vi "TIO RPC Blocking.vi"(8 "error in (no error)":errorcluster, 9 "Payload":string, 10 "Named Method":string="mcu.desc", 11 "TS Connection":T1={"Type"=enum."TCP", "Serial"="serial:///dev/cu.usbserial-00000", "TCP"=refnum, "Timeout"=500}) -> (0 "error out":errorcluster={"status"=TRUE, "code"=-1073807252, "source"="VISA Read in SLIP Decode Serial Read.vi->NN VISA Read.vi->NN RPC.vi"}, 1 "Response":bool, 2 "Respose":string, 3 "TS Connection":T1={"Type"=enum."TCP", "Serial"="serial:///dev/cu.usbserial-00000", "TCP"=refnum, "Timeout"=500})   [LabVIEW 2017]
uses:
  <instrlib>/tio-labview/TIO Library/Socket/TIO Stream Write.vi
  <instrlib>/tio-labview/TIO Library/RPC/RPC Helpers/TIO RPC Form Request.vi
  <instrlib>/tio-labview/TIO Library/Socket/Helpers/TIO Parse Packet.vi
  <instrlib>/tio-labview/TIO Library/Socket/Helpers/TIO SLIP Serial Read.vi
  <instrlib>/tio-labview/TIO Library/Socket/Helpers/TIO SLIP Serial Write.vi
  <instrlib>/tio-labview/TIO Library/Socket/Helpers/TIO Form Packet.vi
  <instrlib>/tio-labview/TIO Library/Socket/Helpers/TIO Serial Checksum CRC32.vi
  <instrlib>/tio-labview/TIO Library/Socket/Helpers/TIO SLIP Encode.vi
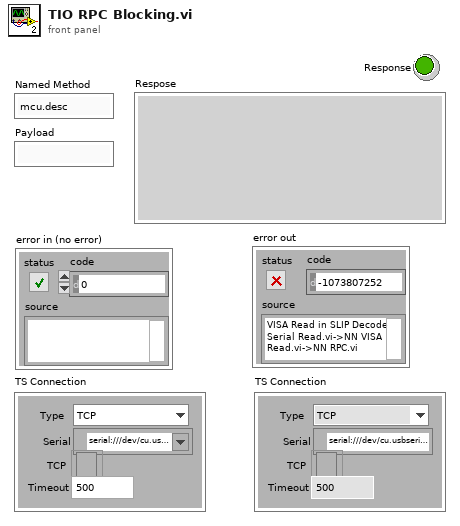
[diagram p1: front panel]
types:
  T1 = cluster{"Type":enum16{"TCP", "Serial"}, "Serial":refnum<visa-resource-name>, "TCP":refnum<k5>, "Timeout":u32}
  T2 = enum8{"Invalid", "Log", "RPC Request", "RPC Reply", "RPC Error", "Stream Description", "User"}
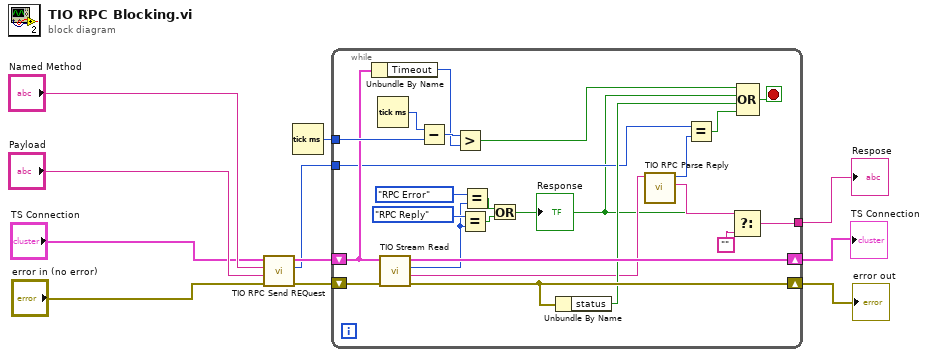
[diagram p0: block diagram]
diagram:
  n1 = call <instrlib>:"TIO RPC Send REQuest.vi"("error in (no error)"="error in (no error)", "Payload"="Payload", "Topic"="Named Method", "TS Connection"="TS Connection") -> ("error out"=w11:errorcluster, "Request ID"=w1:u16, "TS Connection"=w9:T1)  [unwired: 5 in]
  n2 = Tick Count (ms)() -> (millisecond timer value=w6:u32)
  n3 = while {
    shift-right: [w30] -> w10
    shift-left: w11 -> [w35]
    shift-right: [w34] -> w3
    shift-left: w9 -> [w26]
    tunnel: w6 -> [w32]
    tunnel: [w23] -> w2
    tunnel: w1 -> [w21]
    stop <- w27 stop-if-true
    n4 = Unbundle By Name(w26) -> ("Timeout"=w25:u32)
    n5 = Tick Count (ms)() -> (millisecond timer value=w33:u32)
    n6 = call <instrlib>:"TIO Stream Read.vi"("error in (no error)"=w35, "TS Connection"=w26) -> ("error out"=w30:errorcluster, "Payload"=w19:string, "Type"=w15:T2, "TS Connection"=w34:T1)  [unwired: 6 in]
    n7 = Subtract(x=w33, y=w32) -> (x-y=w31:u32)
    n8 = Greater?(x=w31, y=w25) -> (0:w29:bool)
    n9 = Equal?(x=T2."RPC Reply" ("Type"), y=w15) -> (x = y?=w13:bool)
    n10 = Equal?(x=T2."RPC Error" ("Type"), y=w15) -> (x = y?=w14:bool)
    n11 = Or(x=w14, y=w13) -> (x .or. y?=w12:bool)
    "Response" <- w12
    n12 = Unbundle By Name(w30) -> ("status"=w28:bool)
    n13 = call <instrlib>:"TIO RPC Parse Reply.vi"("Payload"=w19) -> ("Payload"=w17:string, "Request ID"=w18:u16)  [unwired: 9 in]
    n14 = Equal?(x=w21, y=w18) -> (x = y?=w20:bool)
    n15 = Select(t=w17, s=w12, f="") -> (s? t:f=w23:string)
    n16 = Compound Arithmetic op=OR(w29, w12, w28, w20) -> (w27:bool)
  }
  "error out" <- w10
  "Respose" <- w2
  "TS Connection" <- w3
